vi "line2array.vi"(0 "data-line":string) -> (1 "Sw-Struc":T1, 2 "Cmd-Struc":T2, 3 "data-array":dbl[](array[numeric]) format="%.2g")   [LabVIEW 2011]
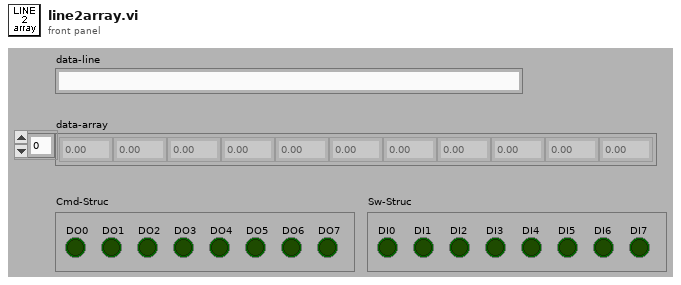
[diagram p1: front panel]
types:
  T1 = cluster{"DI0":bool, "DI1":bool, "DI2":bool, "DI3":bool, "DI4":bool, "DI5":bool, "DI6":bool, "DI7":bool}
  T2 = cluster{"DO0":bool, "DO1":bool, "DO2":bool, "DO3":bool, "DO4":bool, "DO5":bool, "DO6":bool, "DO7":bool}
  T3 = cluster{bool, bool, bool, bool, bool, bool, bool, bool}
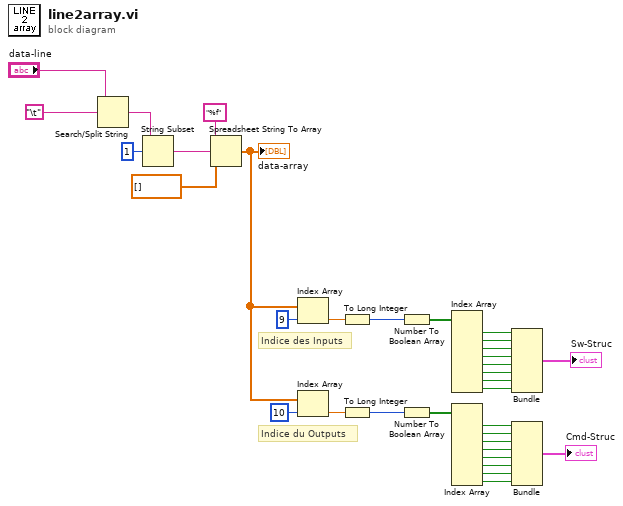
[diagram p0: block diagram]
diagram:
  # "Indice des Inputs"
  # "Indice du Outputs"
  n1 = Search/Split String(string="data-line", search string/char (-)="\t") -> (match + rest of string=w32:string)  [unwired: 1 in, 2 out]
  n2 = String Subset(string=w32, offset (0)=1) -> (substring=w30:string)  [unwired: 1 in]
  n3 = Spreadsheet String To Array(format string="%f", spreadsheet string=w30, array type (2D Dbl)=dbl[] []) -> (array=w2:dbl[])  [unwired: 1 in]
  "data-array" <- w2
  n4 = Index Array(array=w2, index=9) -> (element=w4:dbl)
  n5 = Index Array(array=w2, index=10) -> (element=w26:dbl)
  n6 = To Long Integer(number=w4) -> (32bit integer=w5:i32)
  n7 = To Long Integer(number=w26) -> (32bit integer=w25:i32)
  n8 = Number To Boolean Array(number=w5) -> (Boolean array=w6:bool[])
  n9 = Number To Boolean Array(number=w25) -> (Boolean array=w24:bool[])
  n10 = Index Array(array=w6) -> (element #1=w7:bool, element #2=w8:bool, element #3=w9:bool, element #4=w10:bool, element #5=w11:bool, element #6=w12:bool, element #7=w13:bool, element #8=w14:bool)  [unwired: 8 in]
  n11 = Index Array(array=w24) -> (element #1=w23:bool, element #2=w22:bool, element #3=w21:bool, element #4=w20:bool, element #5=w19:bool, element #6=w18:bool, element #7=w17:bool, element #8=w16:bool)  [unwired: 8 in]
  n12 = Bundle(w7, w8, w9, w10, w11, w12, w13, w14) -> (→"Sw-Struc":T3)  [unwired: 1 in]
  n13 = Bundle(w23, w22, w21, w20, w19, w18, w17, w16) -> (→"Cmd-Struc":T3)  [unwired: 1 in]
